vi "DataChannelRead.vi"(0 "SR865 in":T2, 2 "DataChannel":T1=2 caption="Data channel" items=["X", "Y", "R", "Theta", "IN1", "IN2", "IN3", "IN4", "OUT1", "OUT2", "XNoise", "YNoise", "Phase", "SineOut", "DCLevel", "IntRefFreq", "ExtRefFreq"], 5 "error in":errorcluster) -> (14 "SR865 out":T2, 16 "Signal":dbl caption="Signal, mV", 19 "error out":errorcluster)   [LabVIEW 2018]
uses:
  SR865.ctl
  DataChannel.ctl
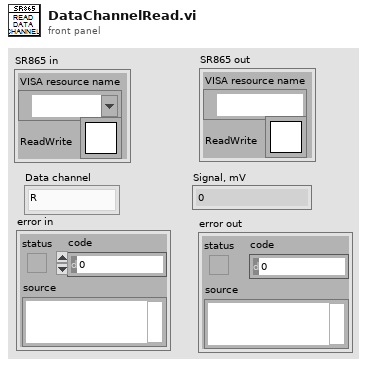
[diagram p1: front panel]
types:
  T1 = typedef "DataChannel.ctl" = u16
  T2 = typedef "SR865.ctl" = cluster{"VISA resource name":refnum<visa-resource-name>, "ReadWrite":T3}
  T3 = typedef "Semaphore RefNum" = refnum<k1>
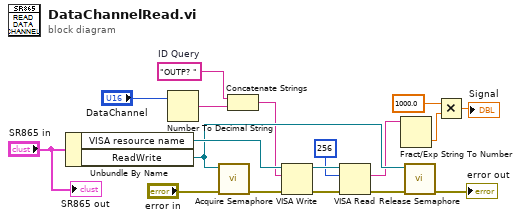
[diagram p0: block diagram]
diagram:
  w7 = "OUTP? "  # ID Query
  n1 = Unbundle By Name("SR865 in") -> ("VISA resource name"=w14:refnum<visa-resource-name>, "ReadWrite"=w9:T3)
  n2 = Number To Decimal String(number="DataChannel") -> (decimal integer string=w4:string)  [unwired: 1 in]
  n3 = call <vilib>:"Acquire Semaphore.vi"("error in (no error)"="error in", "semaphore"=w9) -> ("error out"=w13:errorcluster)  [unwired: 3 in, 2 out]
  n4 = Concatenate Strings(w7, w4) -> (w6:string)
  n5 = VISA Write(VISA resource name=w14, write buffer=w6, error in (no error)=w13) -> (VISA resource name out=w17:refnum<visa-resource-name>, error out=w16:errorcluster)  [unwired: 1 out]
  n6 = VISA Read(VISA resource name=w17, byte count=u32 256, error in (no error)=w16) -> (read buffer=w8:string, error out=w11:errorcluster)  [unwired: 2 out]
  n7 = Fract/Exp String To Number(string=w8) -> (number=w3:dbl)  [unwired: 3 in, 1 out]
  n8 = call <vilib>:"Release Semaphore.vi"("error in (no error)"=w11, "semaphore"=w9) -> ("error out"=→"error out":errorcluster)  [unwired: 4 in, 1 out]
  n9 = Multiply(x=1000.0, y=w3) -> (x*y=→"Signal":dbl)
  "SR865 out" <- "SR865 in"
